vi "Set_Gain_DLPVA-100-BLN-S.vi"(3 "error in":errorcluster, 4 "Status":i32, 5 "Gain [dB]":enum16{"40 dB", "60 dB", "80 dB", "100 dB"}(ring), 6 "index":i32) -> (0 "error out":errorcluster, 1 "Status_out":i32, 2 "index_out":i32)   [LabVIEW 2010, in "FEMTO_LUCI-10.lvlib"]
uses:
  <userlib>/FEMTO/FEMTO_LUCI-10.lvlib
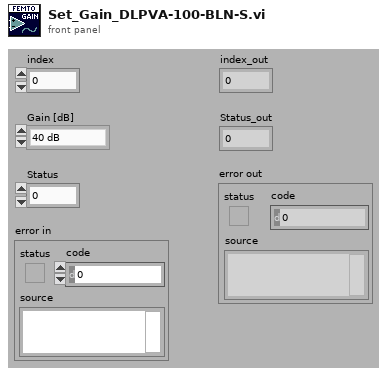
[diagram p1: front panel]
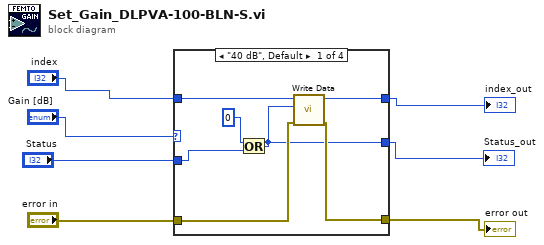
[diagram p0: block diagram]
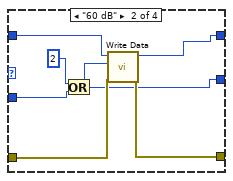
[diagram p2: hidden frame]
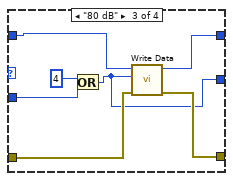
[diagram p3: hidden frame]
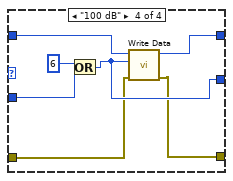
[diagram p4: hidden frame]
diagram:
  n1 = case shown="\"40 dB\", Default" "Gain [dB]" {
    tunnel: "index" -> [w14 w20 w27 w34]
    tunnel: [w13 w19 w26 w33] -> w5
    tunnel: "error in" -> [w12 w17 w24 w30]
    tunnel: [w11 w16 w25 w29] -> w3
    tunnel: "Status" -> [w9 w18 w23 w31]
    tunnel: [w8 w15 w22 w32] -> w1
    frame "40 dB", Default {
      n2 = Or(x=0 ("data_low"), y=w9) -> (x .or. y?=w8:i32)
      n3 = call <userlib>:"Write Data.vi"("error in (no error)"=w12, "data_low"=w8, "index"=w14) -> ("error out"=w11:errorcluster, "index_out"=w13:i32)  [unwired: 1 in, 6 out]
    }
    frame "60 dB" {
      n4 = Or(x=2 ("data_low"), y=w18) -> (x .or. y?=w15:i32)
      n5 = call <userlib>:"Write Data.vi"("error in (no error)"=w17, "data_low"=w15, "index"=w20) -> ("error out"=w16:errorcluster, "index_out"=w19:i32)  [unwired: 1 in, 6 out]
    }
    frame "80 dB" {
      n6 = Or(x=4 ("data_low"), y=w23) -> (x .or. y?=w22:i32)
      n7 = call <userlib>:"Write Data.vi"("error in (no error)"=w24, "data_low"=w22, "index"=w27) -> ("error out"=w25:errorcluster, "index_out"=w26:i32)  [unwired: 1 in, 6 out]
    }
    frame "100 dB" {
      n8 = Or(x=6 ("data_low"), y=w31) -> (x .or. y?=w32:i32)
      n9 = call <userlib>:"Write Data.vi"("error in (no error)"=w30, "data_low"=w32, "index"=w34) -> ("error out"=w29:errorcluster, "index_out"=w33:i32)  [unwired: 1 in, 6 out]
    }
  }
  "index_out" <- w5
  "error out" <- w3
  "Status_out" <- w1
